vi "scaling_calculator.vi"(0 "x1":dbl, 1 "y1":dbl, 2 "x":dbl, 3 "x2":dbl, 4 "y2":dbl) -> (6 "y":dbl)   [LabVIEW 2017]
uses:
  <vilib>/express/express arith-compare/Formula/XNode/ExpressFormulaBlockNode.xnode
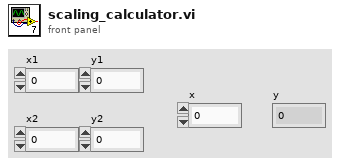
[diagram p1: front panel]
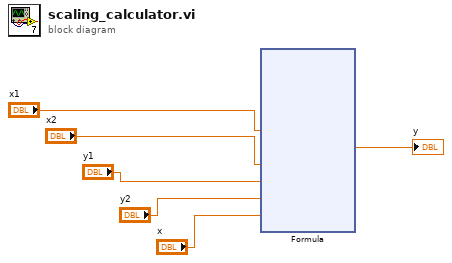
[diagram p0: block diagram]
diagram:
  n1 = xnode "Formula"("X1"="x1", "X2"="x2", "Y1"="y1", "Y2"="y2", "X3"="x") -> ("Result"=→"y":dbl)  [unwired: 1 in, 1 out]
